vi "punto de canto de pajaros labview.vi"() -> ()   [LabVIEW 2017]
uses:
  <vilib>/express/express analysis/Spectral/Block/exnSpectralBlock spectral measurements peak poly.vi
  <vilib>/express/express analysis/Spectral/Block/exnSpectralBlock spectral measurements peak WFM.vi
  <vilib>/express/express analysis/Spectral/XNode/ExpressSpectralMeasurementsBlockNode.xnode
panel:
  out "concatenated string":string
  out "Waveform Graph":dbl[](graph)
  out "size(s) 2":i32
  out "size(s)":i32
  out "Array":dbl[](array[numeric])
  out "Array 3":dbl[](array[numeric])
  out "max value":dbl
  out "Waveform Chart":waveform(dbl)(graph)
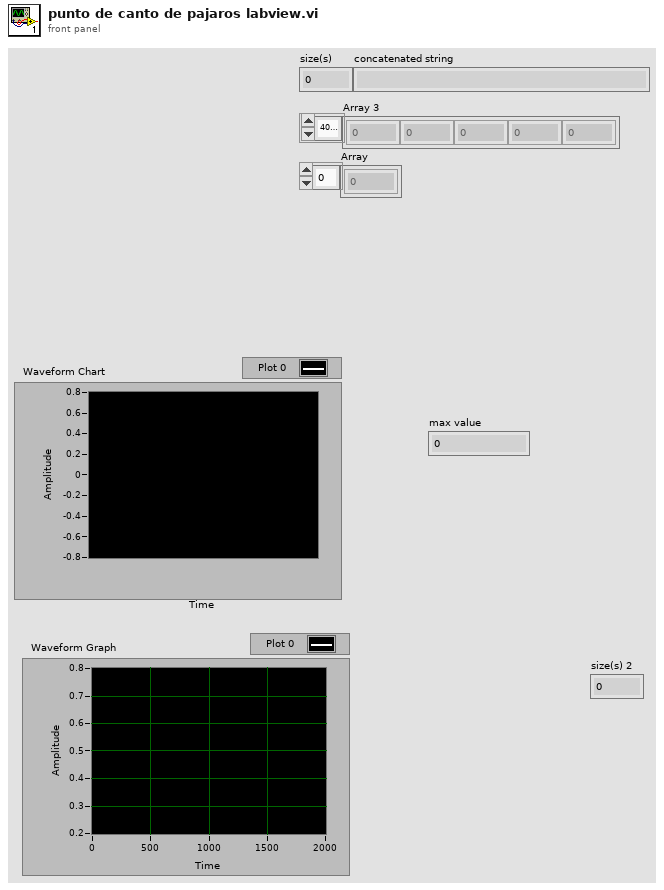
[diagram p1: front panel]
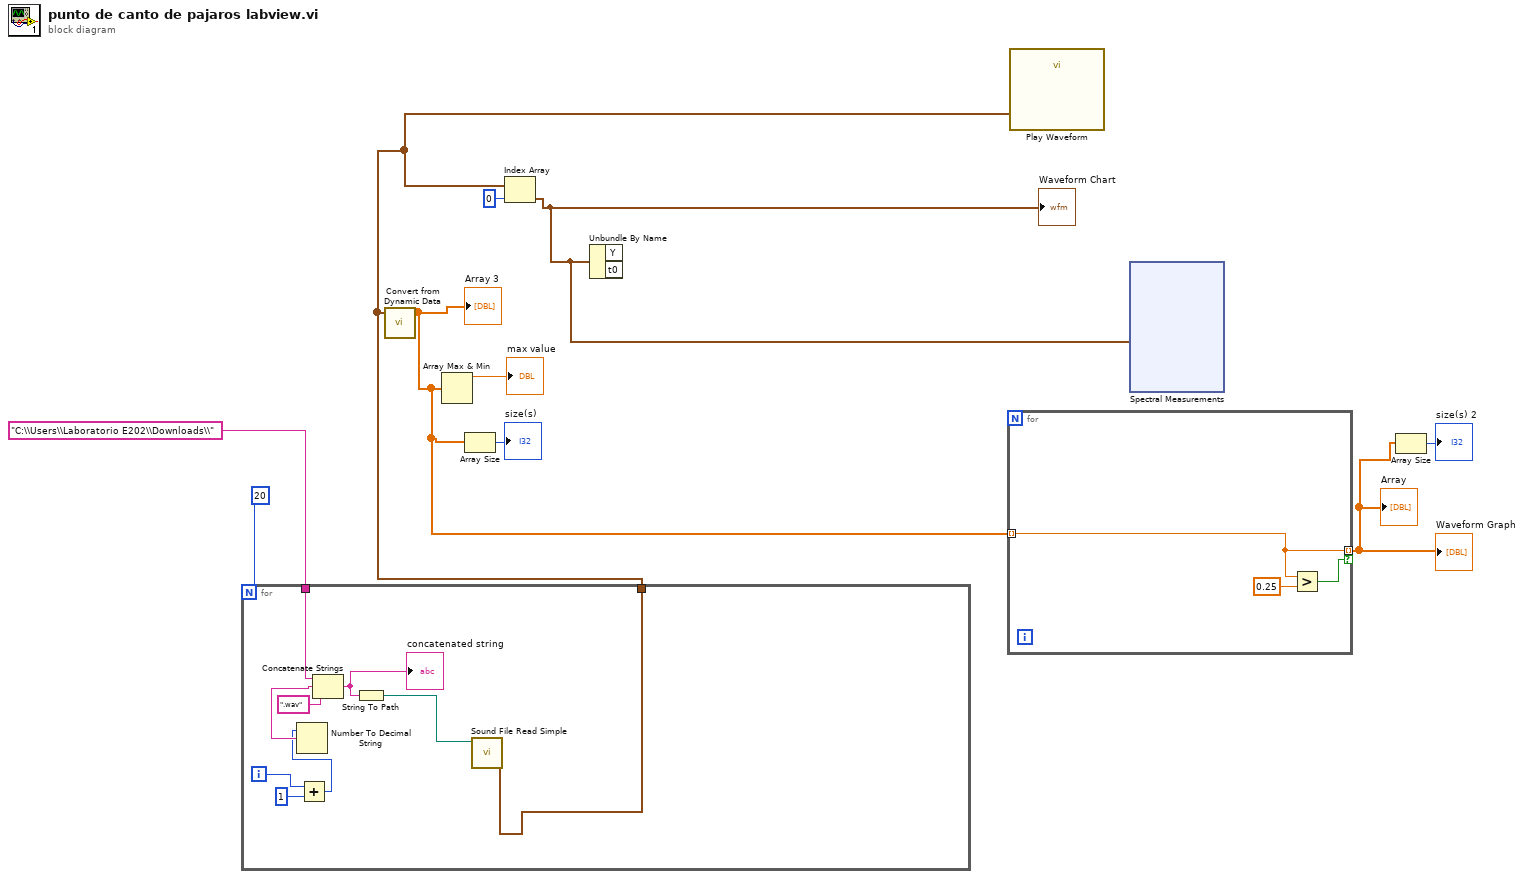
[diagram p0: block diagram]
diagram:
  n1 = for {
    N: 20 -> [_]
    tunnel: "C:\\Users\\Laboratorio E202\\Downloads\\" -> [w19]
    tunnel: [w14] -> w1
    i -> [w13]
    n2 = Add(x=w13, y=1) -> (x+y=w11:i32)
    n3 = Number To Decimal String(number=w11) -> (decimal integer string=w18:string)  [unwired: 1 in]
    n4 = Concatenate Strings(w19, w18, ".wav") -> (w16:string)
    "concatenated string" <- w16
    n5 = String To Path(string=w16) -> (path=w15:path)
    n6 = call <vilib>:"Sound File Read Simple.vi"("path"=w15) -> ("data"=w14:waveform(dbl)[])  [unwired: 7 in, 3 out]
  }
  n7 = call "Convert from Dynamic Data"("Dynamic Data Type"=w1) -> ("Array"=w7:dbl[])  [unwired: 3 in]
  "Array 3" <- w7
  n8 = Array Max & Min(array=w7) -> (max value=→"max value":dbl)  [unwired: 3 out]
  n9 = Array Size(array=w7) -> (size(s)=→"size(s)":i32)
  n10 = Index Array(array=w1, index=0) -> (element=w9:waveform(dbl))
  "Waveform Chart" <- w9
  n11 = Unbundle By Name(w9) -> ()  [unwired: 2 out]
  n12 = for {
    tunnel: [w21] -> w4 mode=indexing if=w20
    tunnel: w7 -> [w21] mode=indexing
    n13 = Greater?(x=w21, y=0.25) -> (0:w20:bool)
  }
  "Array" <- w4
  "Waveform Graph" <- w4
  n14 = call "Play Waveform"("Data"=w1) -> ()  [unwired: 18 in, 1 out]
  n15 = xnode "Spectral Measurements"("Signals"=w9) -> ()  [unwired: 1 in, 3 out]
  n16 = Array Size(array=w4) -> (size(s)=→"size(s) 2":i32)
